vi "sedSpectrometer_logEvent_measuredSpectrum.vi"(8 "error in (no error)":errorcluster, 11 "logevent_measuredSpectrum_Ctl":T1={"imageName"="", "wavelength[2047]"=array[2047 elements], "intensity[2047]"=array[2047 elements], "integrationTime"=0.0, "temperature"=0.0, "priority"=0}) -> (0 "error out":errorcluster, 2 "function return":i32, 3 "logevent_measuredSpectrum_Ctl out":T1)   [LabVIEW 2016, in "SALLV_sedSpectrometer.lvlib"]
doc: "int sedSpectrometer_shm_logEvent_measuredSpectrumLV(sedSpectrometer_logevent_measuredSpectrumLV *logevent_measuredSpectrum_Ctl );"
uses:
  SALLV_sedSpectrometer.lvlib
  DataTypes/logevent_measuredSpectrum.ctl
  SALLV_sedSpectrometer.so
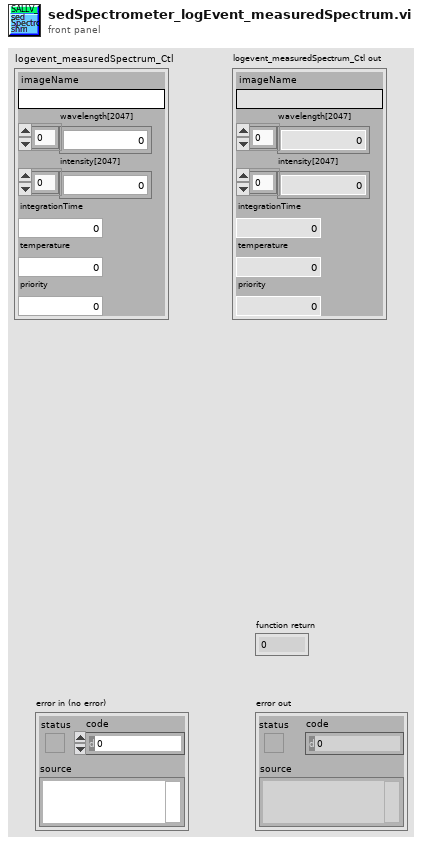
[diagram p1: front panel]
types:
  T1 = typedef "SALLV_sedSpectrometer.lvlib/logevent_measuredSpectrum.ctl" = cluster{"imageName":string, "wavelength[2047]":dbl[], "intensity[2047]":dbl[], "integrationTime":sgl, "temperature":dbl, "priority":i32}
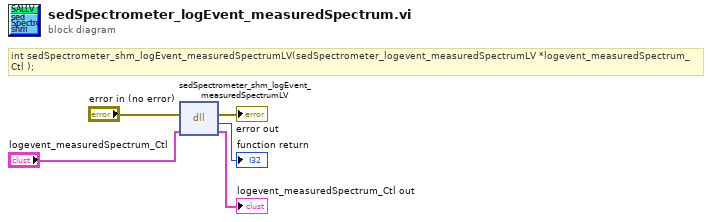
[diagram p0: block diagram]
diagram:
  # "int sedSpectrometer_shm_logEvent_measuredSpectrumLV(sedSpectrometer_logevent_measuredSpectrumLV *logevent_measuredSpectrum_Ctl );"
  n1 = dll-call lib="home/harini/TCS/ts_sallv_sedSpectrometer_371/SALLV_sedSpectrometer.*" fn="sedSpectrometer_shm_logEvent_measuredSpectrumLV"(error in="error in (no error)", "logevent_measuredSpectrum_Ctl"="logevent_measuredSpectrum_Ctl") -> (error out=→"error out":errorcluster, →"function return":i32, "logevent_measuredSpectrum_Ctl"=→"logevent_measuredSpectrum_Ctl out":T1)  [unwired: 2 in, 1 out]
